vi "Write VoltageToILCDAC.vi"(10 "VoltageToILCDAC":refnum<class "VoltageToILCDACRaw.lvclass">, 11 "ILCControlledActuatorCylinder in":refnum<class "ILCControlledActuatorCylinder.lvclass">) -> (3 "ILCControlledActuatorCylinder out":refnum<class "ILCControlledActuatorCylinder.lvclass">)   [LabVIEW 2015, in "ILCControlledActuatorCylinder.lvclass"]
uses:
  ILCControlledActuatorCylinder.lvclass
  Calculators/VoltageToILCDACRaw/VoltageToILCDACRaw.lvclass
  ILCControlledActuatorCylinder.lvclass/ILCControlledActuatorCylinder.ctl
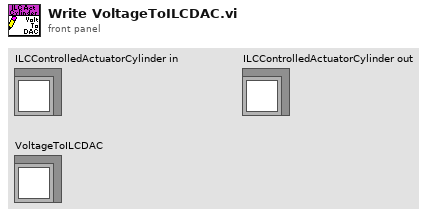
[diagram p1: front panel]
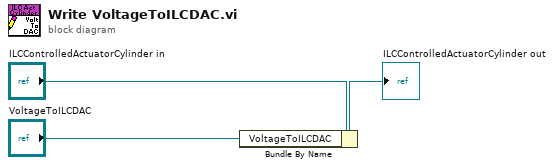
[diagram p0: block diagram]
diagram:
  n1 = Bundle By Name(cluster="ILCControlledActuatorCylinder in", "VoltageToILCDAC"="VoltageToILCDAC") -> (→"ILCControlledActuatorCylinder out":refnum<class "ILCControlledActuatorCylinder.lvclass">)
